vi "RMS.vi"(11 "Filtered X":dbl[](array[numeric])) -> (1 "RMS2>RMS1":dynamicdata(graph), 2 "RMS1":dynamicdata(graph), 3 "RMS2":dynamicdata(graph), 4 "rms value 2":dbl, 5 "rms value":dbl)   [LabVIEW 2021]
uses:
  <vilib>/ptbypt/NI_PtbyPt.lvlib
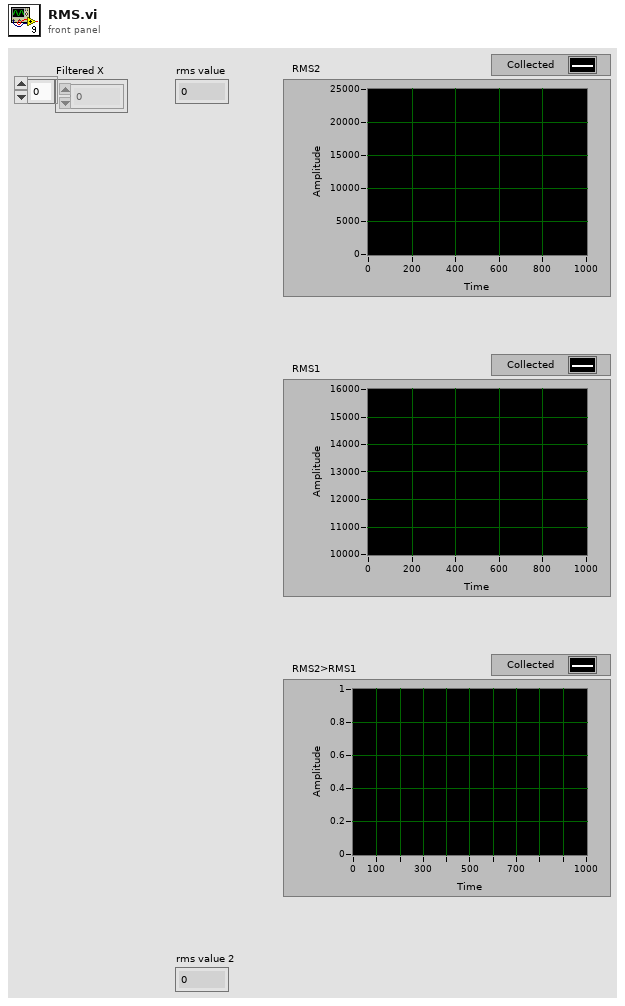
[diagram p1: front panel]
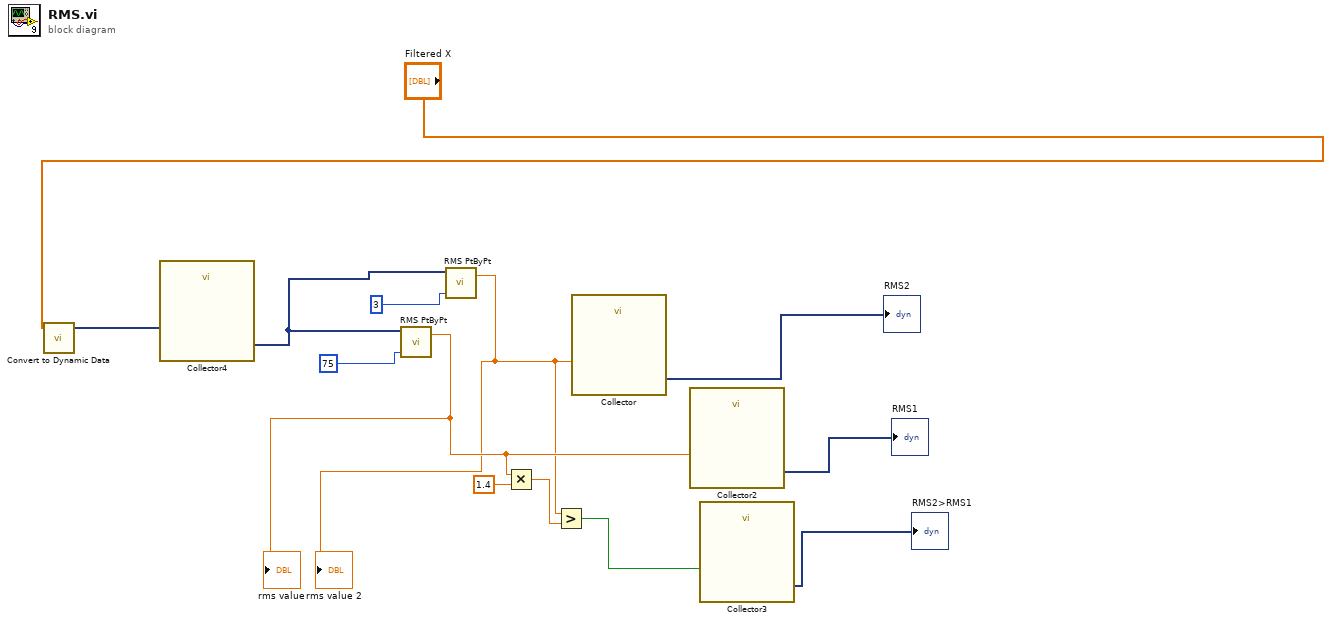
[diagram p0: block diagram]
diagram:
  n1 = call "Convert to Dynamic Data"("Array"="Filtered X") -> ("Dynamic Data Type"=w9:dynamicdata)  [unwired: 3 in]
  n2 = call "Collector4"("Signals"=w9) -> ("Collected Signals"=w10:dynamicdata)  [unwired: 9 in, 1 out]
  n3 = call <vilib>:"RMS PtByPt.vi"("sample length"=75, "x"=w10) -> ("rms value"=w12:dbl)  [unwired: 2 in, 1 out]
  "rms value" <- w12
  n4 = call <vilib>:"RMS PtByPt.vi"("sample length"=3, "x"=w10) -> ("rms value"=w11:dbl)  [unwired: 2 in, 1 out]
  "rms value 2" <- w11
  n5 = Multiply(x=w12, y=1.4) -> (x*y=w6:dbl)
  n6 = Greater?(x=w11, y=w6) -> (0:w7:bool)
  n7 = call "Collector"("Signals"=w11) -> ("Collected Signals"=→"RMS2":dynamicdata)  [unwired: 9 in, 1 out]
  n8 = call "Collector2"("Signals"=w12) -> ("Collected Signals"=→"RMS1":dynamicdata)  [unwired: 9 in, 1 out]
  n9 = call "Collector3"("Signals"=w7) -> ("Collected Signals"=→"RMS2>RMS1":dynamicdata)  [unwired: 9 in, 1 out]
